vi "LinearFilter_ResetToValue.vi"(9 "InputValue":dbl, 11 "In LINEAR_FILTER":T1 {"Outputs" format="%13.5p"; "Inputs" format="%13.5p"; "OutputGains" format="%13.5p"; "InputGains" format="%13.5p"}) -> (3 "Out LINEAR_FILTER":T1 {"Outputs" format="%13.5p"; "Inputs" format="%13.5p"; "OutputGains" format="%13.5p"; "InputGains" format="%13.5p"})   [LabVIEW 2019, in "Trajectory_Library.lvlib"]
doc: "Reset the filter state. Sets the saved inputs and outputs to \"InputValue:\"\n\n\nInputs: \n - inLinearfilter - Linear filter data structure\n - InputValue - This value is used to fill the saved input and output values\n\nOutputs:\n - outLinearfilter - Updated linear filter data structurea"
uses:
  Trajectory_Library.lvlib
  LINEAR_FILTER.ctl
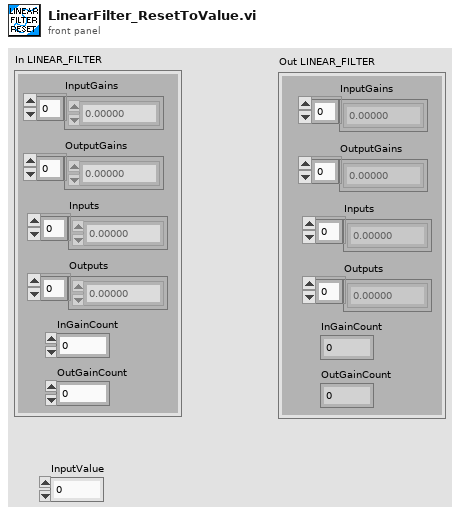
[diagram p1: front panel]
types:
  T1 = typedef "Trajectory_Library.lvlib/LINEAR_FILTER.ctl" = cluster{"InputGains":dbl[], "OutputGains":dbl[], "Inputs":dbl[], "Outputs":dbl[], "InGainCount":i32, "OutGainCount":i32}
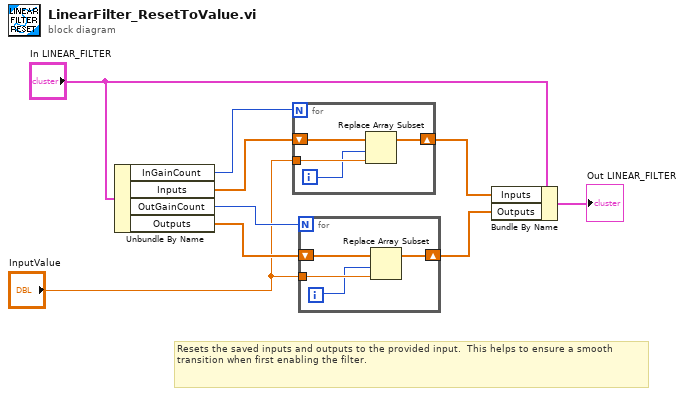
[diagram p0: block diagram]
diagram:
  # "Resets the saved inputs and outputs to the provided input.  This helps to ensure a smooth\ntransition when first enabling the filter."
  n1 = Unbundle By Name("In LINEAR_FILTER") -> ("InGainCount"=w3:i32, "Inputs"=w7:dbl[], "OutGainCount"=w2:i32, "Outputs"=w4:dbl[])
  n2 = for {
    N: w3 -> [_]
    shift-right: [w12] -> w6
    shift-left: w7 -> [w13]
    tunnel: "InputValue" -> [w11]
    i -> [w10]
    n3 = Replace Array Subset(array=w13, new element=w11, index=w10) -> (w12:dbl[])
  }
  n4 = for {
    N: w2 -> [_]
    shift-right: [w16] -> w5
    shift-left: w4 -> [w17]
    tunnel: "InputValue" -> [w15]
    i -> [w14]
    n5 = Replace Array Subset(array=w17, new element=w15, index=w14) -> (w16:dbl[])
  }
  n6 = Bundle By Name(cluster="In LINEAR_FILTER", "Inputs"=w6, "Outputs"=w5) -> (→"Out LINEAR_FILTER":T1)
